vi "old_vi_Wait.vi"(0 "Data Task in":refnum<k21>, 5 "data task error in":errorcluster, 7 "#DAQ outputs (1-13)":i32, 9 "PS VISA in":refnum<visa-resource-name>, 11 "PS error in":errorcluster caption="PS error in (no error)", 12 "Wait Filepath":path=path "C:/Users/ga11/Desktop/VI/results/3PtestChrgRest.lvm" caption="Filename", 13 "Wait time":dbl) -> (4 "data task out":refnum<k21>, 6 "data task error out":errorcluster, 10 "PS Visa Out":refnum<visa-resource-name>, 15 "PS error out":errorcluster)   [LabVIEW 2025]
uses:
  Battery-Testing-Software-NHR/system_development/v0.1/Drivers-NHR-9200/NHR/Public/Data/Read (Ave Current).vi
  Battery-Testing-Software-NHR/system_development/v0.1/Drivers-NHR-9200/NHR/Public/Data/Low Level/Fetch (Ave Voltage).vi
  Battery-Testing-Software-NHR/system_development/v0.1/Drivers-Essentials/NH Research Regenerative Test Series.lvlib
panel:
  out "Ave Current (A)":dbl
  out "Ave Voltage (V)":dbl
  out "WaitElapsed Time (s)":i32 caption="Elapsed Time (s)"
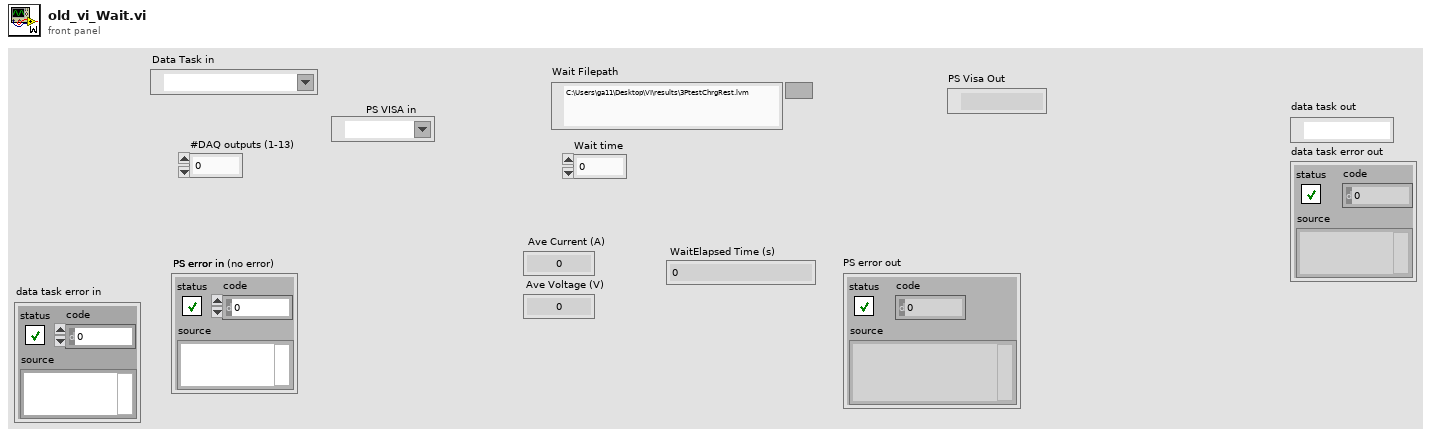
[diagram p1: front panel]
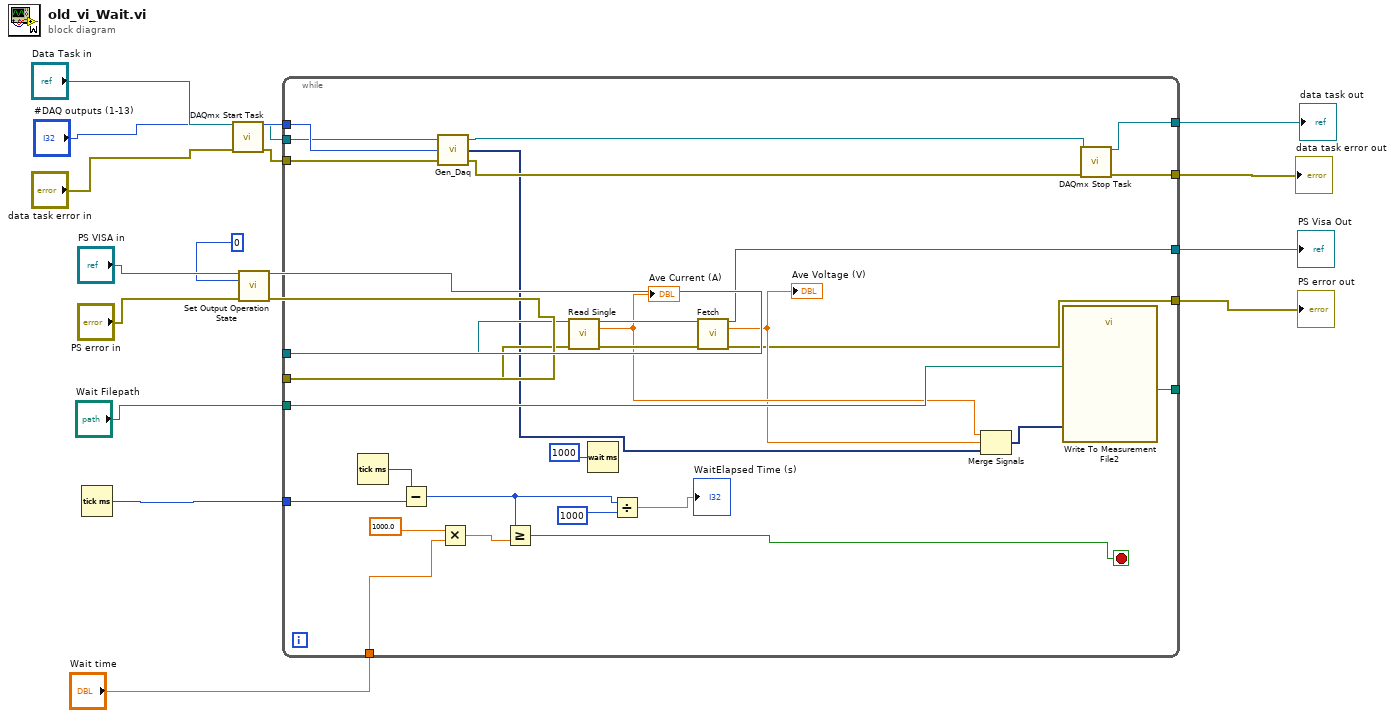
[diagram p0: block diagram]
diagram:
  n1 = Tick Count (ms)() -> (millisecond timer value=w16:u32)
  n2 = call <vilib>:"DAQmx Start Task.vi"("task/channels in"="Data Task in", "error in"="data task error in") -> ("task out"=w2:refnum<k21>, "error out"=w1:errorcluster)  [unwired: 12 in]
  n3 = call "Set Output Operation State.vi"("VISA resource name"="PS VISA in", "Mode (0: Off)"=0, "error in (no error)"="PS error in") -> ("VISA resource name out"=w4:refnum<visa-resource-name>, "error out"=w3:errorcluster)  [unwired: 11 in]
  n4 = while {
    tunnel: w4 -> [w44]
    tunnel: w3 -> [w43]
    tunnel: "Wait time" -> [w39]
    tunnel: [w36] -> _
    tunnel: w16 -> [w35]
    tunnel: "Wait Filepath" -> [w34]
    tunnel: [w27] -> w12
    tunnel: [w26] -> w11
    tunnel: "#DAQ outputs (1-13)" -> [w23]
    tunnel: w2 -> [w22]
    tunnel: w1 -> [w21]
    tunnel: [w20] -> w7
    tunnel: [w19] -> w6
    stop <- w40 stop-if-true
    n5 = Tick Count (ms)() -> (millisecond timer value=w41:u32)
    n6 = Subtract(x=w41, y=w35) -> (x-y=w33:u32)
    n7 = call "Gen_Daq.vi"("error in"=w21, "#DAQ outputs (1-13)"=w23, "task/channels in"=w22) -> ("error out"=w24:errorcluster, "DaQ_output"=w18:dynamicdata, "task out"=w25:refnum<k21>)
    n8 = Multiply(x=1000.0, y=w39) -> (x*y=w37:dbl)
    n9 = Greater Or Equal?(x=w33, y=w37) -> (x >= y?=w40:bool)
    n10 = call-poly "Read Single.vi"("VISA resource name"=w44, "error in (no error)"=w43) -> ("VISA resource name out"=w45:refnum<visa-resource-name>, "Ave Current (A)"=w30:dbl, "error out"=w46:errorcluster)  [unwired: 11 in]
    "Ave Current (A)" <- w30
    n11 = Wait (ms)(milliseconds to wait=1000) -> ()  [unwired: 1 out]
    n12 = Divide(x=w33, y=1000) -> (x/y=→"WaitElapsed Time (s)":dbl)
    n13 = call-poly "Fetch.vi"("VISA resource name"=w45, "error in (no error)"=w46) -> ("VISA resource name out"=w27:refnum<visa-resource-name>, "Ave Voltage (V)"=w28:dbl, "error out"=w26:errorcluster)  [unwired: 11 in]
    "Ave Voltage (V)" <- w28
    n14 = Merge Signals "Merge Signals"(w30, w28, w18) -> (w29:dynamicdata)
    n15 = call "Write To Measurement File2"("Signals"=w29, "Filename"=w34) -> ("Filename Out"=w36:path)  [unwired: 15 in, 2 out]
    n16 = call <vilib>:"DAQmx Stop Task.vi"("task/channels in"=w25, "error in"=w24) -> ("task out"=w20:refnum<k21>, "error out"=w19:errorcluster)  [unwired: 12 in]
  }
  "PS Visa Out" <- w12
  "PS error out" <- w11
  "data task out" <- w7
  "data task error out" <- w6
